vi "Set Constant Label.vi"(8 "error in (no error)":errorcluster, 9 "QD Combo Box Ref":refnum<vi>, 10 "Shift Not Pressed?":bool, 11 "Constant in":refnum<vi>) -> (0 "error out":errorcluster)   [LabVIEW 2017]
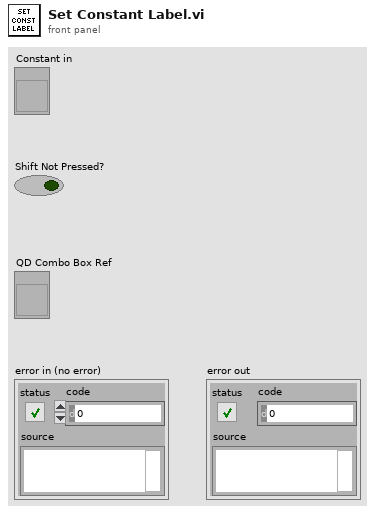
[diagram p1: front panel]
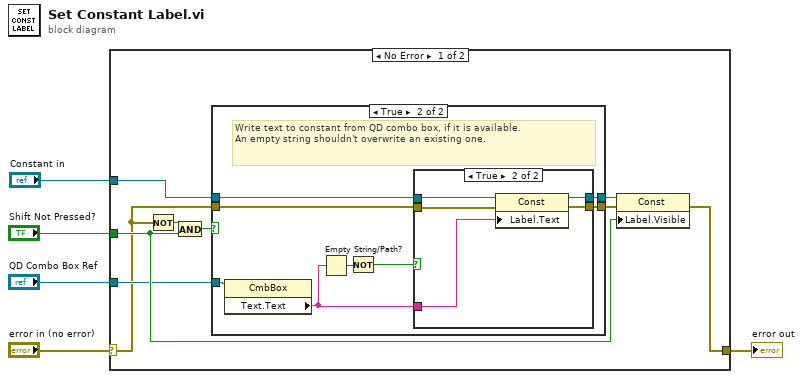
[diagram p0: block diagram]
diagram:
  n1 = case shown="No Error" "error in (no error)" {
    selector: "error in (no error)" -> [w12 w32]
    tunnel: [w7 w32] -> w5
    tunnel: "Shift Not Pressed?" -> [w14 _]
    tunnel: "QD Combo Box Ref" -> [w13 _]
    tunnel: "Constant in" -> [w6 _]
    frame No Error {
      n2 = Not(x=w12) -> (.not. x?=w11:bool)
      n3 = And(x=w11, y=w14) -> (x .and. y?=w10:bool)
      n4 = case shown="True" w10 {
        tunnel: w13 -> [_ w24]
        tunnel: w6 -> [w16 w20]
        tunnel: [w16 w23] -> w8
        tunnel: [w15 w22] -> w9
        tunnel: w12 -> [w15 w21]
        frame False {
        }
        frame True {
          # "Write text to constant from QD combo box, if it is available.\nAn empty string shouldn't overwrite an existing one."
          n5 = property class="CmbBox"(reference=w24) -> ("Text.Text"=w19:string)  [unwired: 1 in, 2 out]
          n6 = Empty String/Path?(string/path=w19) -> (empty?=w17:bool)
          n7 = Not(x=w17) -> (.not. x?=w18:bool)
          n8 = case shown="True" w18 {
            tunnel: [w26 w31] -> w23
            tunnel: [w25 w30] -> w22
            tunnel: w21 -> [w25 w29]
            tunnel: w20 -> [w26 w28]
            tunnel: w19 -> [_ w27]
            frame False {
            }
            frame True {
              n9 = property class="Const"(reference=w28, error in=w29, "Label.Text"=w27) -> (reference out=w31:refnum<vi>, error out=w30:errorcluster)
            }
          }
        }
      }
      n10 = property class="Const"(reference=w8, error in=w9, "Label.Visible"=w14) -> (error out=w7:errorcluster)  [unwired: 1 out]
    }
    frame Error {
    }
  }
  "error out" <- w5
